vi "Actor Core.vi"(8 "error in (no error)":errorcluster, 11 "Parent Actor in":refnum<class "Parent Actor.lvclass">) -> (0 "error out":errorcluster, 3 "Parent Actor out":refnum<class "Parent Actor.lvclass">)   [LabVIEW 2015, in "Parent Actor.lvclass"]
uses:
  Parent Actor.lvclass
  Parent Actor.lvclass/Parent Actor.ctl
  Parent Message/Parent Message.lvclass
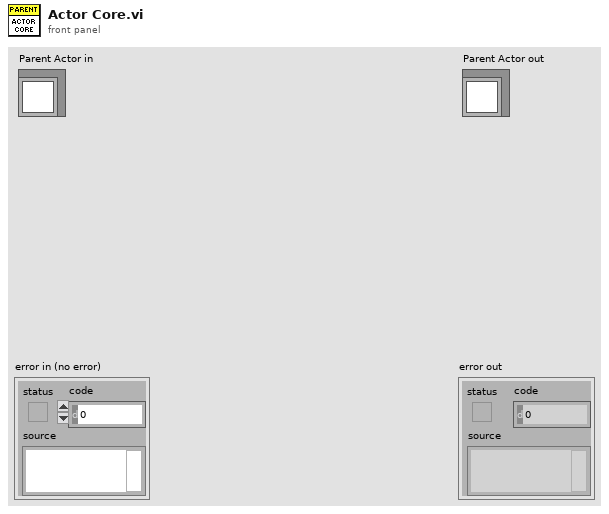
[diagram p1: front panel]
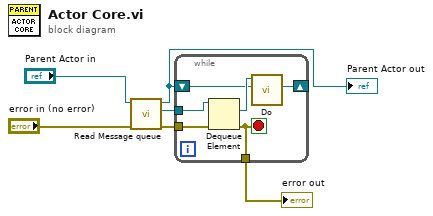
[diagram p0: block diagram]
diagram:
  n1 = call "Read Message queue.vi"("error in (no error)"="error in (no error)", "Parent Actor in"="Parent Actor in") -> ("error out"=w3:errorcluster, "Message queue"=w5:refnum<queue>, "Parent Actor out"=w1:refnum<class "Parent Actor.lvclass">)  [unwired: 7 in]
  "Parent Actor out" <- w1
  n2 = while {
    tunnel: w5 -> [w12]
    shift-right: [w9] -> _
    shift-left: w1 -> [w10]
    tunnel: w3 -> [w8]
    tunnel: [w7] -> w2
    stop <- w7 stop-if-true
    n3 = Dequeue Element(queue=w12, error in (no error)=w8) -> (element=w11:refnum<class "Parent Message.lvclass">, error out=w7:errorcluster)  [unwired: 1 in, 2 out]
    n4 = call-dynamic "Do.vi"("Parent Actor"=w10, "Parent Message in"=w11) -> ("Parent Actor out"=w9:refnum<class "Parent Actor.lvclass">)  [unwired: 7 in, 2 out]
  }
  "error out" <- w2
